vi "LakeShore 340 Heater Range Calc.vi"(3 "Power":dbl format="%.2e", 4 "Heater Range":u32, 5 "Start Control?":bool, 6 "Resistance":dbl format="%.2f") -> (0 "Percent Power Out":dbl, 1 "Command":string, 2 "Heater Range Out":u32)   [LabVIEW 2020]
panel:
  out "Max Range power":dbl format="%.2e"
  out "Range":dbl format="%.2e"
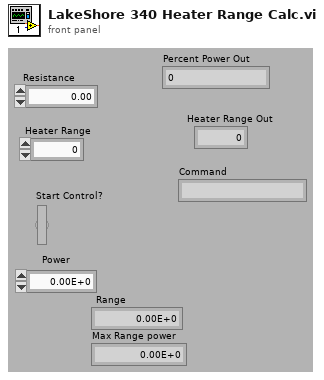
[diagram p1: front panel]
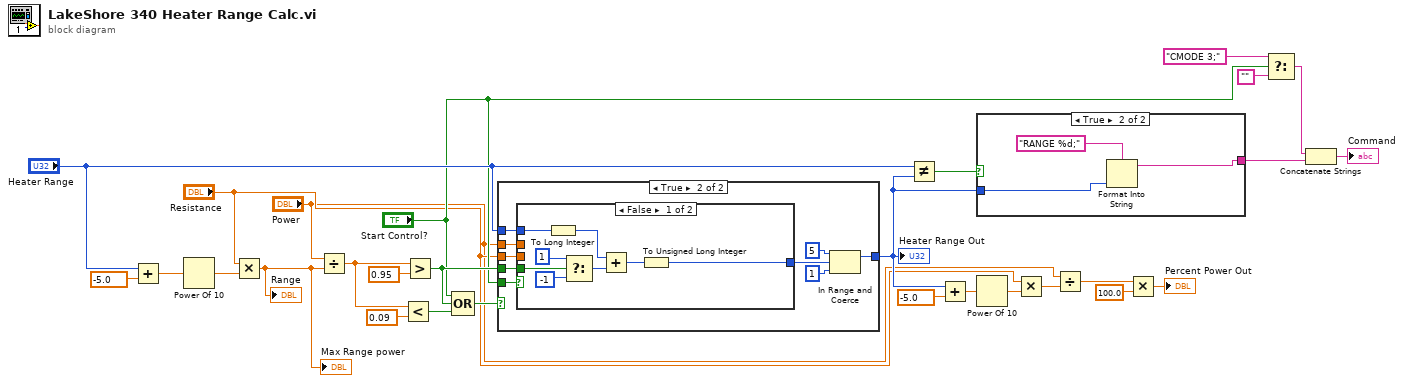
[diagram p0: block diagram]
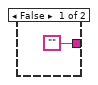
[diagram p2: hidden frame]
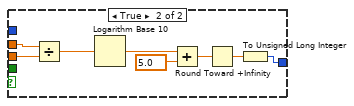
[diagram p4: hidden frame]
diagram:
  n1 = Add(x="Heater Range", y=-5.0) -> (x+y=w14:dbl)
  n2 = Power Of 10(x=w14) -> (10^x=w12:dbl)
  n3 = Multiply(x="Resistance", y=w12) -> (x*y=w11:dbl)
  "Range" <- w11
  "Max Range power" <- w11
  n4 = Divide(x="Power", y=w11) -> (x/y=w24:dbl)
  n5 = Less?(x=w24, y=0.09) -> (x < y?=w20:bool)
  n6 = Greater?(x=w24, y=0.95) -> (0:w18:bool)
  n7 = Compound Arithmetic op=OR("Start Control?", w18, w20) -> (w21:bool)
  n8 = case shown="True" w21 {
    tunnel: "Heater Range" -> [w29 w35]
    tunnel: [w29 w34] -> w7
    tunnel: w18 -> [_ w38]
    tunnel: "Power" -> [_ w32]
    tunnel: "Resistance" -> [_ w31]
    tunnel: "Start Control?" -> [_ w30]
    frame False {
    }
    frame True {
      n9 = case shown="False" w30 {
        tunnel: w38 -> [w46 _]
        tunnel: w35 -> [w43 _]
        tunnel: [w39 w50] -> w33
        tunnel: w32 -> [_ w52]
        tunnel: w31 -> [_ w51]
        frame False {
          n10 = To Long Integer(number=w43) -> (32bit integer=w40:i32)
          n11 = Select(t=1 ("Heater Range"), s=w46, f=-1) -> (s? t:f=w42:i32)
          n12 = Add(x=w40, y=w42) -> (x+y=w41:i32)
          n13 = To Unsigned Long Integer(number=w41) -> (unsigned 32bit integer=w39:u32)
        }
        frame True {
          n14 = Divide(x=w52, y=w51) -> (x/y=w48:dbl)
          n15 = Logarithm Base 10(1:w48) -> (0:w49:dbl)
          n16 = Add(x=w49, y=5.0) -> (x+y=w47:dbl)
          n17 = Round Toward +Infinity(x=w47) -> (ceil(x): smallest int >= x=w53:dbl)
          n18 = To Unsigned Long Integer(number=w53) -> (unsigned 32bit integer=w50:u32)
        }
      }
      n19 = In Range and Coerce(upper limit=u32 5, x=w33, lower limit=u32 1) -> (coerced(x)=w34:u32)  [unwired: 1 out]
    }
  }
  "Heater Range Out" <- w7
  n20 = Not Equal?(x="Heater Range", y=w7) -> (x != y?=w17:bool)
  n21 = Add(x=w7, y=-5.0) -> (x+y=w9:dbl)
  n22 = case shown="True" w17 {
    tunnel: ["" w56] -> w16
    tunnel: w7 -> [_ w58]
    frame False {
    }
    frame True {
      n23 = Format Into String(format string="RANGE %d;", w58) -> (resulting string=w56:string)  [unwired: 2 in, 1 out]
    }
  }
  n24 = Power Of 10(x=w9) -> (10^x=w8:dbl)
  n25 = Multiply(x="Resistance", y=w8) -> (x*y=w5:dbl)
  n26 = Divide(x="Power", y=w5) -> (x/y=w3:dbl)
  n27 = Multiply(x=w3, y=100.0) -> (x*y=→"Percent Power Out":dbl)
  n28 = Select(t="CMODE 3;", s="Start Control?", f="") -> (s? t:f=w26:string)
  n29 = Concatenate Strings(w26, w16) -> (→"Command":string)
